vi "Configure Dialog.vi"(8 "error in (no error)":errorcluster, 11 "Configure RTD [RTD] Msg.lvclass":refnum<class "Configure RTD [RTD] Msg.lvclass">) -> (0 "error out":errorcluster, 2 "Ok?":bool, 3 "Configure RTD [RTD] Msg.lvclass":refnum<class "Configure RTD [RTD] Msg.lvclass">)   [LabVIEW 2015, in "CS++DMM.lvlib" / "Configure RTD [RTD] Msg.lvclass"]
uses:
  Configure RTD [RTD] Msg.lvclass
  Configure RTD [RTD] Msg.lvclass/Configure RTD [RTD] Msg.ctl
panel:
  in  "resistance (0.0 ohms)":dbl
  in  "alpha (0.0)":dbl
  in  "Cancel Button":bool
  in  "OK Button":bool
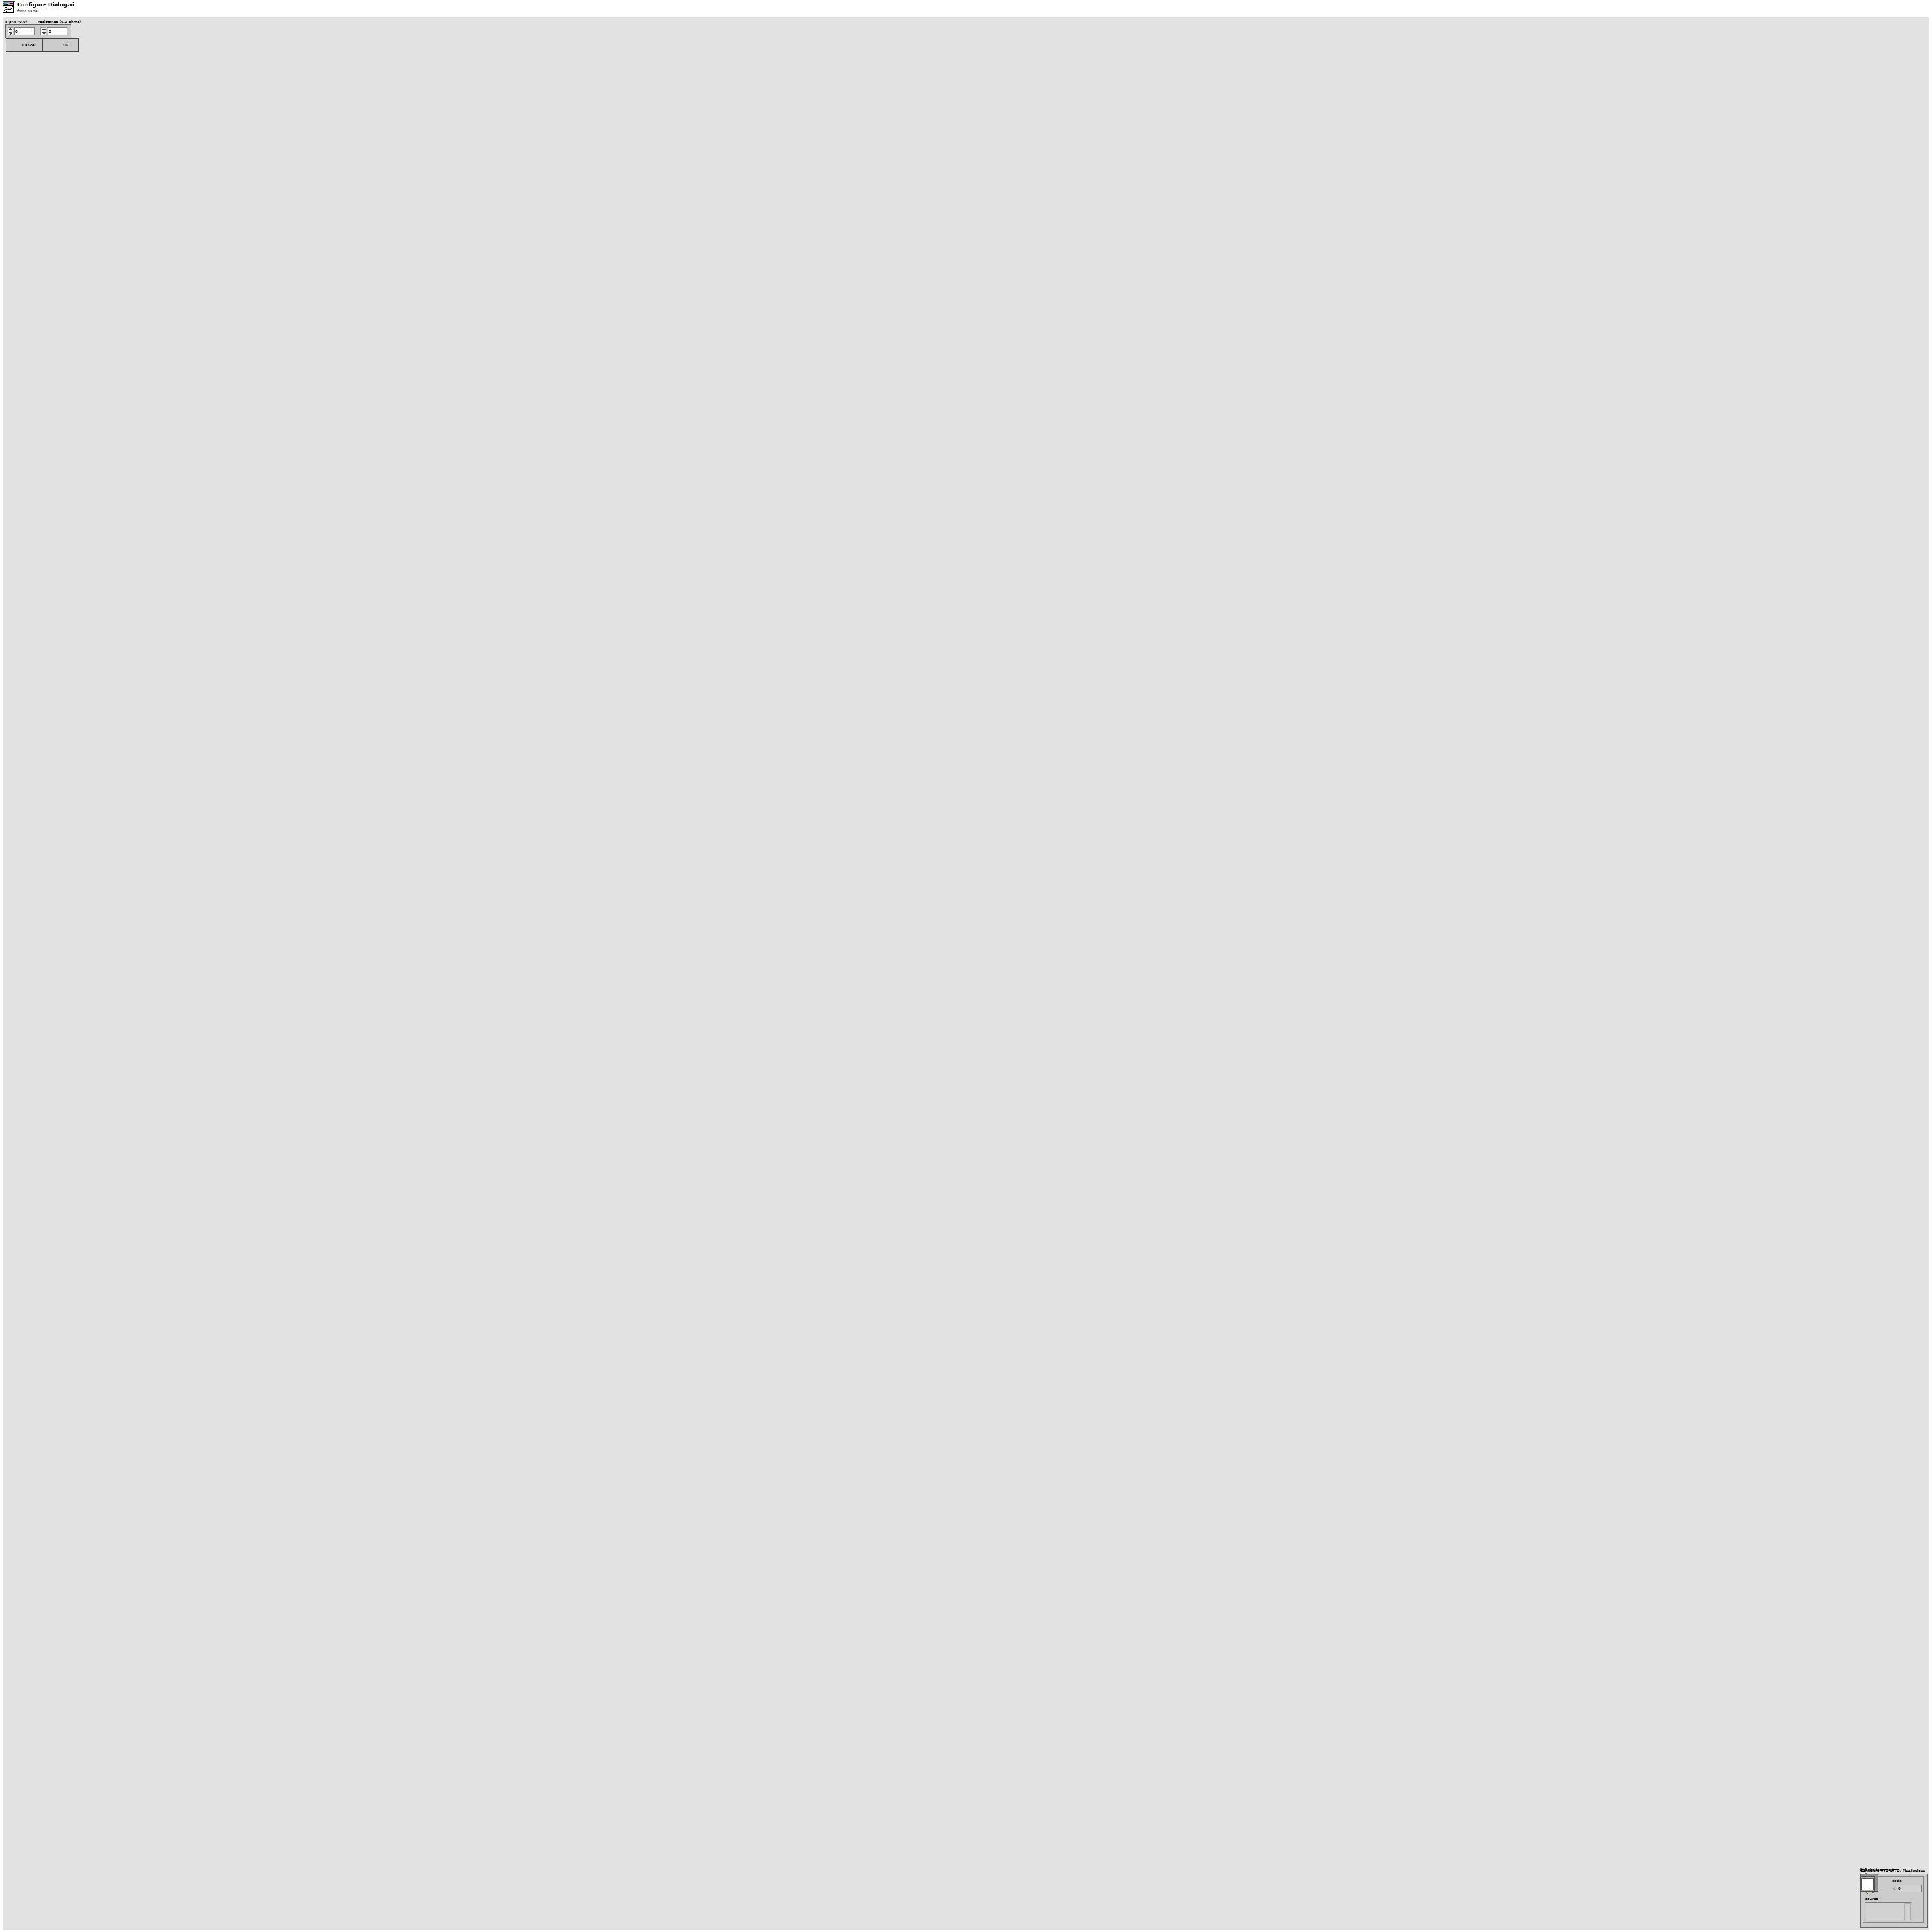
[diagram p1: front panel]
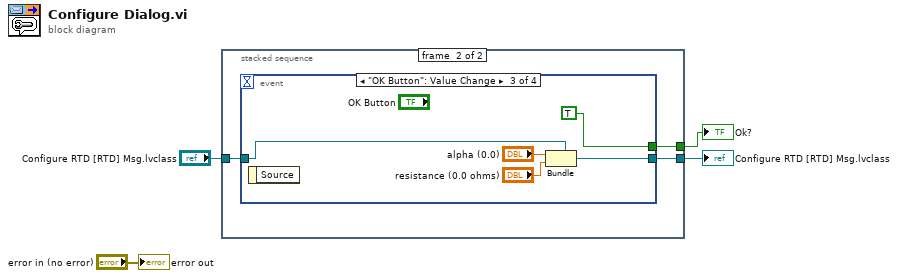
[diagram p0: block diagram]
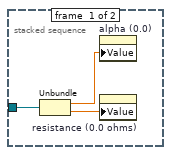
[diagram p2: hidden frame]
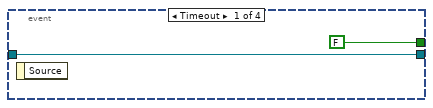
[diagram p3: hidden frame]
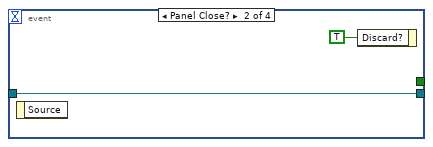
[diagram p4: hidden frame]
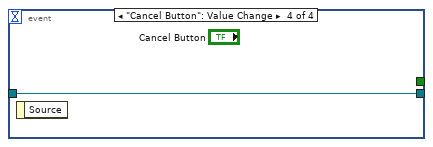
[diagram p5: hidden frame]
diagram:
  n1 = stacked-sequence {
    tunnel: [_ w10] -> w3
    tunnel: [_ w9] -> w2
    tunnel: "Configure RTD [RTD] Msg.lvclass" -> [w7 w8]
    frame #0 {
      n2 = Unbundle ("Seq0Unbundler")(w7) -> (w6:dbl, w5:dbl)
      n3 = property on="alpha (0.0)" class="DigNum (strict)"("Value"=w6) -> ()  [unwired: 2 in, 2 out]
      n4 = property on="resistance (0.0 ohms)" class="DigNum (strict)"("Value"=w5) -> ()  [unwired: 2 in, 2 out]
    }
    frame #1 {
      n5 = event shown="[2] \"OK Button\": Value Change" {
        selector: _ -> [_ _ _ _]
        dyn-events: _ -> [_ _ _ _]
        timeout: _ -> [_ _ _ _]
        tunnel: [w11 w13 w17 w20] -> w9
        tunnel: w8 -> [w11 w13 w19 w20]
        tunnel: [FALSE _ TRUE _] -> w10
        event Timeout {
          n6 = event-data() -> ()  [unwired: 1 in, 1 out]
        }
        event Panel Close? {
          n7 = event-data() -> ()  [unwired: 1 in, 1 out]
          n8 = event-data ("Event Filter Node")("Discard?"=TRUE) -> ()  [unwired: 1 in, 1 out]
        }
        event "OK Button": Value Change {
          n9 = event-data() -> ()  [unwired: 1 in, 1 out]
          n10 = Bundle ("Main-Bundler")(cluster=w19, "alpha (0.0)", "resistance (0.0 ohms)") -> (w17:refnum<class "Configure RTD [RTD] Msg.lvclass">)
        }
        event "Cancel Button": Value Change {
          n11 = event-data() -> ()  [unwired: 1 in, 1 out]
        }
      }
    }
  }
  "Ok?" <- w3
  "Configure RTD [RTD] Msg.lvclass" <- w2
  "error out" <- "error in (no error)"
